vi "Drop Through Click.vi"(8 "error in (no error)":errorcluster, 11 "hwnd":u32) -> (0 "error out":errorcluster)   [LabVIEW 2016, in "LV MDI.lvclass"]
uses:
  LV MDI.lvclass
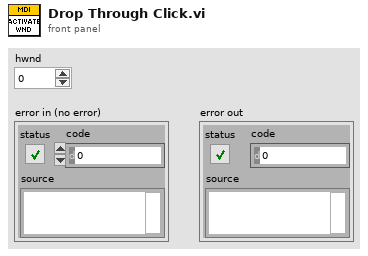
[diagram p1: front panel]
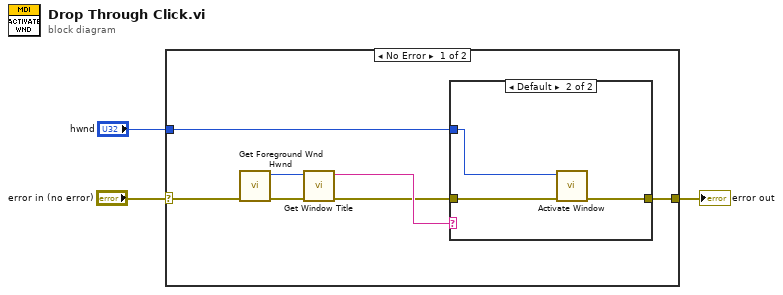
[diagram p0: block diagram]
diagram:
  n1 = case shown="No Error" "error in (no error)" {
    selector: "error in (no error)" -> [w8 w15]
    tunnel: [w5 w15] -> w2
    tunnel: "hwnd" -> [w4 _]
    frame No Error {
      n2 = call "Get Foreground Wnd Hwnd.vi"("error in (no error)"=w8) -> ("error out"=w7:errorcluster, "hwnd"=w6:u32)  [unwired: 9 in]
      n3 = call "Get Window Title.vi"("error in (no error)"=w7, "hwnd"=w6) -> ("error out"=w9:errorcluster, "Window Title"=w10:string)  [unwired: 8 in]
      n4 = case shown="Default" w10 {
        tunnel: w4 -> [_ w14]
        tunnel: [w11 w13] -> w5
        tunnel: w9 -> [w11 w12]
        frame "Open" {
        }
        frame Default {
          n5 = call "Activate Window.vi"("error in (no error)"=w12, "Hwnd"=w14) -> ("error out"=w13:errorcluster)  [unwired: 9 in]
        }
      }
    }
    frame Error {
    }
  }
  "error out" <- w2
